vi "readRawData.vi"(8 "ErrorIn":errorcluster, 10 "I2C Ref In":T1={"myRIO Reference"={"myRIO Model"=enum."Unknown", "myRIO Hardware Reference"={"Generic FPGA Reference"=refnum, "Allow multiple opens"=FALSE}}, "I2C Channels Enum"=enum."Not Connected", "I2C Configuration"={"I2C Transfer Rate"=enum."Fast mode (400 kbps)"}}, 11 "QueuesIn":T9) -> (0 "ErrorOut":errorcluster, 1 "RawAccelerationData":u8[](array[numeric]), 2 "I2C Ref Out":T1={"myRIO Reference"={"myRIO Model"=enum."Unknown", "myRIO Hardware Reference"={"Generic FPGA Reference"=refnum, "Allow multiple opens"=FALSE}}, "I2C Channels Enum"=enum."Not Connected", "I2C Configuration"={"I2C Transfer Rate"=enum."Fast mode (400 kbps)"}}, 3 "QueuesOut":T9)   [LabVIEW 2019]
uses:
  utilities/Queues.ctl
  UIVIs/UIInput.ctl
  UIVIs/UIOutput.ctl
  UIVIs/AccelerationDataFrames.ctl
  <vilib>/myRIO/Instrument Drivers/Onboard IO/I2C/typedefs/I2C Reference.ctl
  <vilib>/myRIO/Common/Instrument Driver Framework/Utilities/typedefs/myRIO Generic Hardware Reference.ctl
  <vilib>/myRIO/Common/Instrument Driver Framework/Utilities/typedefs/Hardware Version Enum.ctl
  <vilib>/myRIO/Common/Instrument Driver Framework/Utilities/typedefs/myRIO v1.0 Reference.ctl
  <vilib>/myRIO/Common/Instrument Driver Framework/Utilities/typedefs/Generic FPGA Reference.ctl
  <vilib>/myRIO/Common/Instrument Driver Framework/myRIO v1.0/I2C/typedefs/I2C Channels Enum.ctl
  <vilib>/myRIO/Instrument Drivers/Onboard IO/I2C/typedefs/I2C Configuration.ctl
  <vilib>/myRIO/Instrument Drivers/Onboard IO/I2C/typedefs/I2C Transfer Rate.ctl
  <vilib>/Utility/error.llb/Error Cluster From Error Code.vi
  <vilib>/myRIO/Common/Instrument Driver Framework/myRIO v1.0/I2C/vis/myRIO v1.0 Write I2C.vi
  <vilib>/myRIO/Common/Instrument Driver Framework/myRIO v1.0/I2C/vis/myRIO v1.0 Read I2C.vi
  <vilib>/myRIO/Instrument Drivers/Onboard IO/I2C/I2C.lvlib
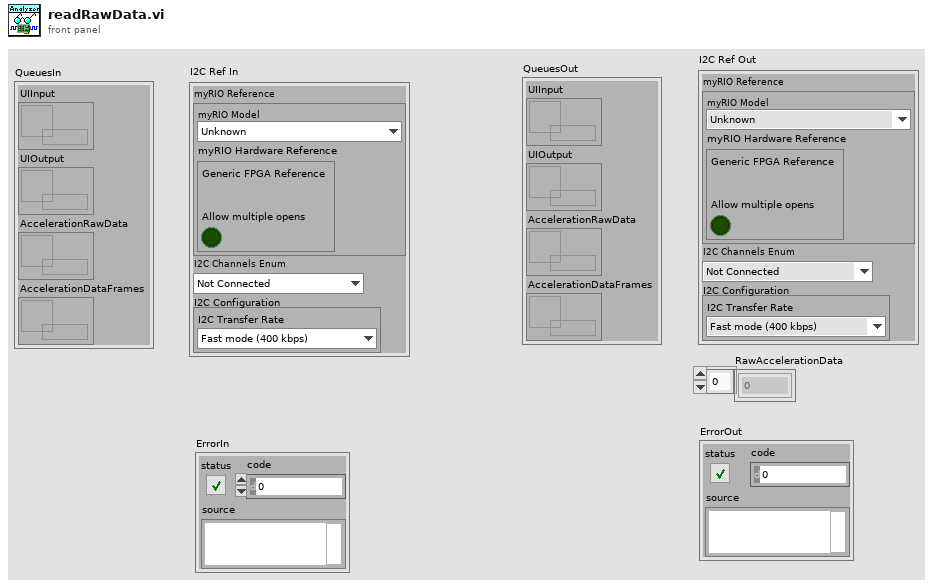
[diagram p1: front panel]
types:
  T1 = typedef "I2C.lvlib/I2C Reference.ctl" = cluster{"myRIO Reference":T2, "I2C Channels Enum":T6, "I2C Configuration":T7}
  T2 = typedef "myRIO Generic Hardware Reference.ctl" = cluster{"myRIO Model":T3, "myRIO Hardware Reference":T4}
  T3 = typedef "Hardware Version Enum.ctl" = enum16{"Unknown", "myRIO-1900", "myRIO-1950", "roboRIO", "NI ELVIS RIO CM", "ELVIS III"}
  T4 = typedef "myRIO v1.0 Reference.ctl" = cluster{"Generic FPGA Reference":T5, "Allow multiple opens":bool}
  T5 = typedef "Generic FPGA Reference.ctl" = refnum<k20>
  T6 = typedef "I2C Channels Enum.ctl" = enum16{"Not Connected", "A/I2C", "B/I2C", "I2C/I2C"}
  T7 = typedef "I2C.lvlib/I2C Configuration.ctl" = cluster{"I2C Transfer Rate":T8}
  T8 = typedef "I2C.lvlib/I2C Transfer Rate.ctl" = enum16{"Standard mode (100 kbps)", "Fast mode (400 kbps)"}
  T9 = typedef "Queues.ctl" = cluster{"UIInput":refnum<queue>, "UIOutput":refnum<queue>, "AccelerationRawData":refnum<queue>, "AccelerationDataFrames":refnum<queue>}
  T10 = typedef "UIOutput.ctl" = cluster{"Aquiring data":bool, "CriticalError":errorcluster, "InternalError":errorcluster, "FIFO overflow":bool, "Analyzing data":bool, "Device working":bool}
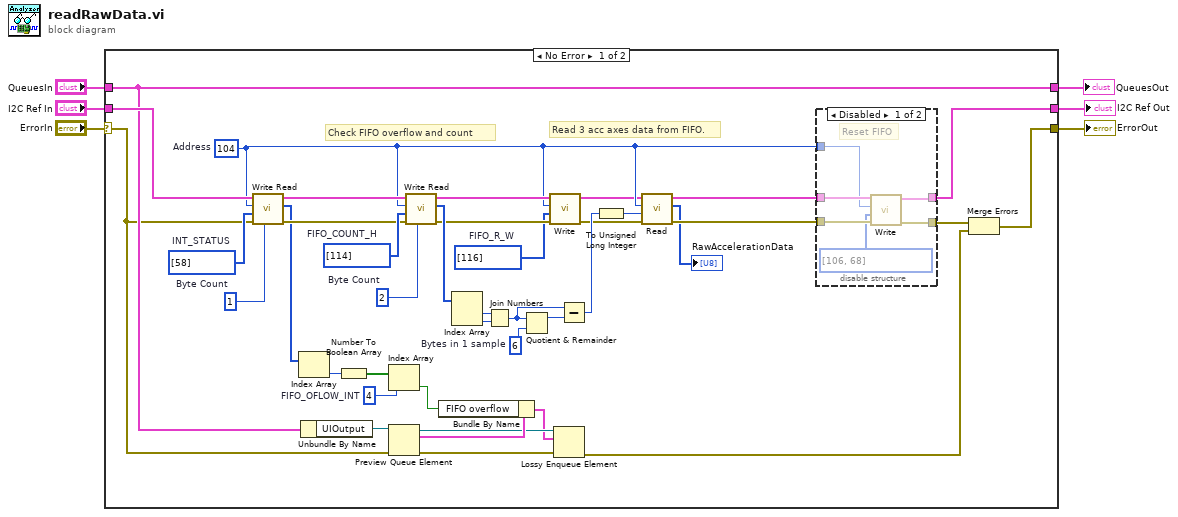
[diagram p0: block diagram]
diagram:
  n1 = case shown="No Error" "ErrorIn" {
    selector: "ErrorIn" -> [w30 w57]
    tunnel: [w23 w57] -> w5
    tunnel: "I2C Ref In" -> [w41 w56]
    tunnel: "QueuesIn" -> [w32 w55]
    tunnel: [w32 w55] -> w2
    tunnel: [w7 w56] -> w1
    frame No Error {
      w12 = u8[] [116]  # FIFO_R_W
      w34 = 4  # FIFO_OFLOW_INT
      w37 = u32 1  # Byte Count
      w38 = u8[] [58]  # INT_STATUS
      w42 = u16 6  # Bytes in 1 sample
      w45 = u8[] [114]  # FIFO_COUNT_H
      w11 = u8 104  # Address
      w46 = u32 2  # Byte Count
      # "Check FIFO overflow and count"
      # "Read 3 acc axes data from FIFO."
      n2 = call <vilib>:"Write Read.vi"("Byte Count"=w37, "error in (no error)"=w30, "Bytes to Write"=w38, "Slave Address (7-bit)"=w11, "I2C Ref In"=w41) -> ("error out"=w39:errorcluster, "Bytes Read"=w33:u8[], "I2C Ref Out"=w40:T1)  [unwired: 3 in]
      n3 = Index Array(array=w33) -> (element=w36:u8)  [unwired: 1 in]
      n4 = Unbundle By Name(w32) -> ("UIOutput"=w31:refnum<queue>)
      n5 = Number To Boolean Array(number=w36) -> (Boolean array=w35:bool[])
      n6 = Index Array(array=w35, index=w34) -> (element=w28:bool)
      n7 = Preview Queue Element(queue=w31, error in (no error)=w30) -> (queue out=w27:refnum<queue>, element=w29:T10, error out=w26:errorcluster)  [unwired: 1 in, 1 out]
      n8 = call <vilib>:"Write Read.vi"("Byte Count"=w46, "error in (no error)"=w39, "Bytes to Write"=w45, "Slave Address (7-bit)"=w11, "I2C Ref In"=w40) -> ("error out"=w13:errorcluster, "Bytes Read"=w44:u8[], "I2C Ref Out"=w14:T1)  [unwired: 3 in]
      n9 = Bundle By Name(cluster=w29, "FIFO overflow"=w28) -> (w25:T10)
      n10 = Index Array(array=w44) -> (element #1=w43:u8, element #2=w17:u8)  [unwired: 2 in]
      n11 = Join Numbers(hi=w43, lo=w17) -> ((hi.lo)=w21:u16)
      n12 = Quotient & Remainder(x=w21, y=w42) -> (x-y*floor(x/y)=w22:u16)  [unwired: 1 out]
      n13 = call <vilib>:"Write.vi"("error in (no error)"=w13, "Bytes to Write"=w12, "Slave Address (7-bit)"=w11, "I2C Ref In"=w14) -> ("error out"=w10:errorcluster, "I2C Ref Out"=w9:T1)  [unwired: 6 in]
      n14 = Lossy Enqueue Element(queue=w27, element=w25, error in (no error)=w26) -> (error out=w24:errorcluster)  [unwired: 3 out]
      n15 = Subtract(x=w21, y=w22) -> (x-y=w20:u16)
      n16 = To Unsigned Long Integer(number=w20) -> (unsigned 32bit integer=w8:u32)
      n17 = call <vilib>:"Read.vi"("error in (no error)"=w10, "Byte Count"=w8, "Slave Address (7-bit)"=w11, "I2C Ref In"=w9) -> ("error out"=w19:errorcluster, "Bytes Read"=→"RawAccelerationData":u8[], "I2C Ref Out"=w18:T1)  [unwired: 4 in]
      n18 = disable-structure shown="Disabled" {
        disable-tunnel: w19 -> [w52 w53]
        disable-tunnel: w18 -> [w50 w54]
        disable-tunnel: [w47 w54] -> w7
        disable-tunnel: [w49 w53] -> w15
        disable-tunnel: w11 -> [w48 _]
        frame Disabled {
          # "Reset FIFO"
          n19 = call <vilib>:"Write.vi"("error in (no error)"=w52, "Bytes to Write"=u8[] [106, 68], "Slave Address (7-bit)"=w48, "I2C Ref In"=w50) -> ("error out"=w49:errorcluster, "I2C Ref Out"=w47:T1)  [unwired: 6 in]
        }
        frame Enabled {
        }
      }
      n20 = Merge Errors(w15, w24) -> (w23:errorcluster)
    }
    frame Error {
    }
  }
  "ErrorOut" <- w5
  "QueuesOut" <- w2
  "I2C Ref Out" <- w1
